vi "Launch_Async_Email.vi"() -> (0 "error out":errorcluster)   [LabVIEW 2018]
uses:
  Globals/Constants_global.vi
  Email_transfer_global.vi
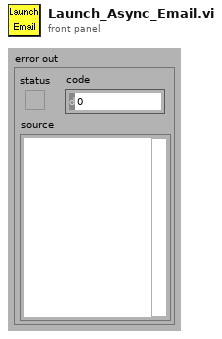
[diagram p1: front panel]
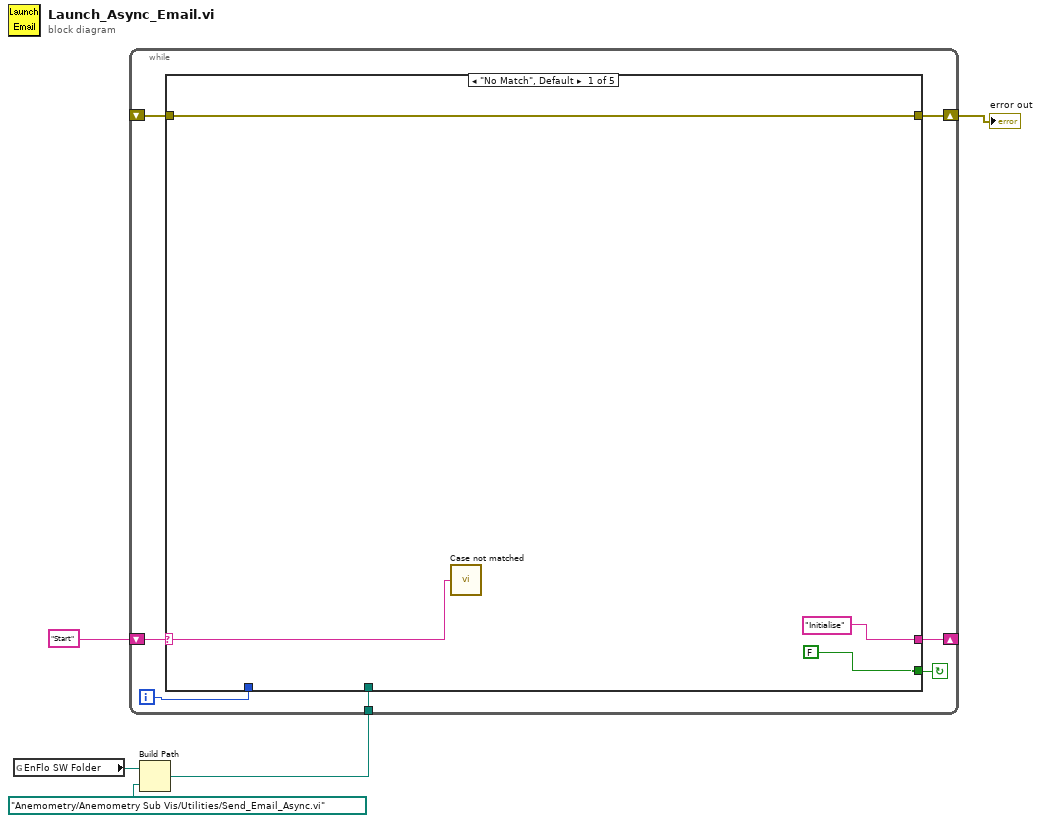
[diagram p0: block diagram]
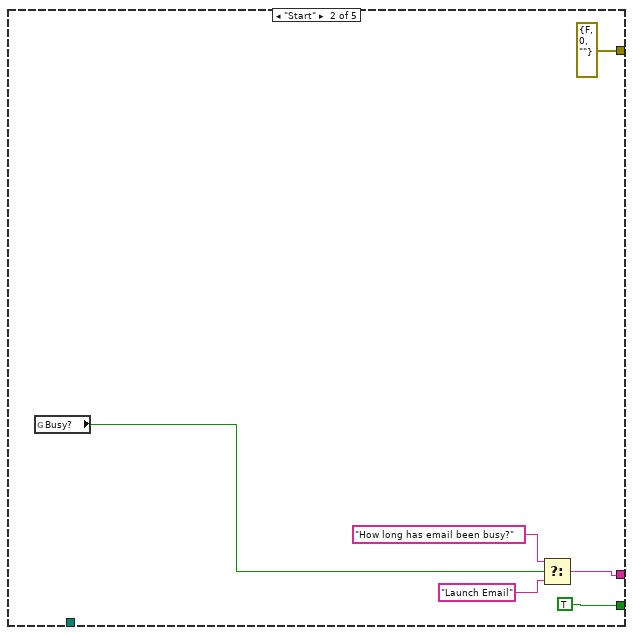
[diagram p2: hidden frame]
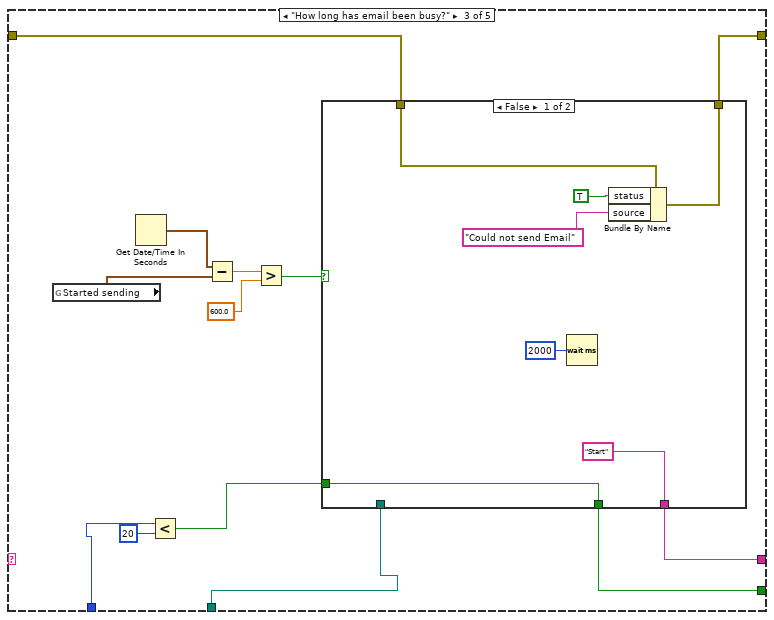
[diagram p3: hidden frame]
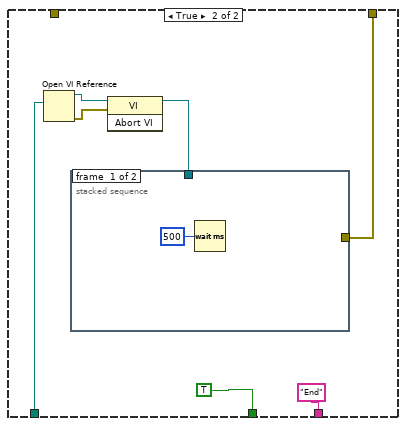
[diagram p4: hidden frame]
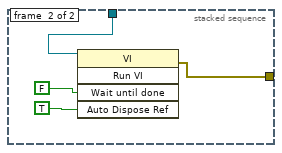
[diagram p5: hidden frame]
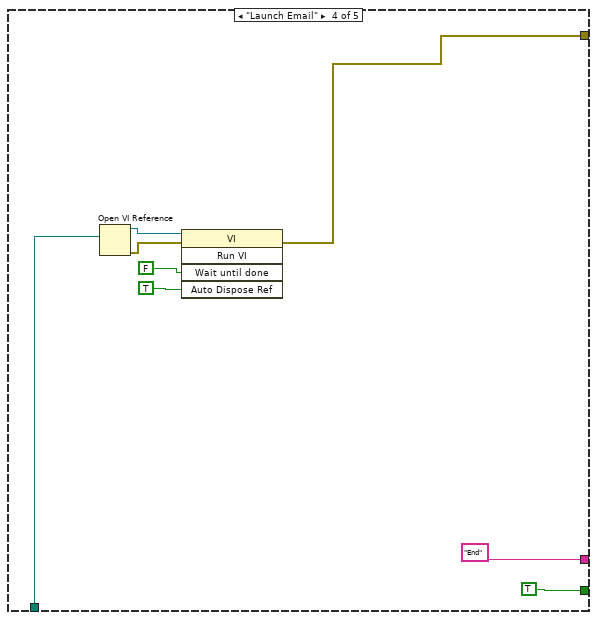
[diagram p6: hidden frame]
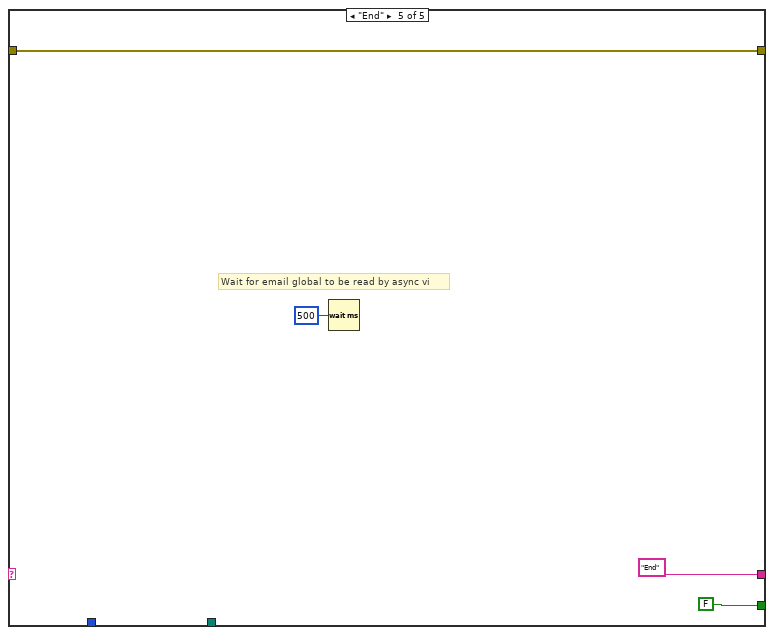
[diagram p7: hidden frame]
diagram:
  n1 = global read "Constants_global.vi" "EnFlo SW Folder"() -> (w3:path)
  n2 = Build Path(base path=w3, name or relative path=path "Anemometry/Anemometry Sub Vis/Utilities/Send_Email_Async.vi") -> (appended path=w2:path)
  n3 = while {
    shift-left: "Start" -> [w10]
    shift-right: [w11] -> _
    tunnel: w2 -> [w9]
    shift-right: [w8] -> w1
    shift-left: _ -> [w7]
    i -> [w6]
    stop <- w12 continue-if-true
    n4 = case shown="\"No Match\", Default" w10 {
      selector: w10 -> [w13 _ _ _ _]
      tunnel: [FALSE TRUE w28 TRUE FALSE] -> w12
      tunnel: ["Initialise" w18 w29 "End" "End"] -> w11
      tunnel: w9 -> [_ _ w30 w56 _]
      tunnel: [w14 errorcluster {"status"=FALSE, "code"=0, "source"=""} ("error out") w24 w55 w63] -> w8
      tunnel: w7 -> [w14 _ w23 _ w63]
      tunnel: w6 -> [_ _ w27 _ _]
      frame "No Match", Default {
        n5 = call "Case not matched.vi"("Case Name not Matched"=w13) -> ()
      }
      frame "Start" {
        n6 = global read "Email_transfer_global.vi" "Busy?"() -> (w20:bool)
        n7 = Select(t="How long has email been busy?", s=w20, f="Launch Email") -> (s? t:f=w18:string)
      }
      frame "How long has email been busy?" {
        n8 = global read "Email_transfer_global.vi" "Started sending"() -> (w34:timestamp)
        n9 = Get Date/Time In Seconds() -> (seconds since 1Jan1904=w35:timestamp)
        n10 = Less?(x=w27, y=20) -> (x < y?=w25:bool)
        n11 = Subtract(x=w35, y=w34) -> (x-y=w33:dbl)
        n12 = Greater?(x=w33, y=600.0) -> (0:w31:bool)
        n13 = case shown="False" w31 {
          tunnel: w30 -> [_ w47]
          tunnel: ["Start" "End"] -> w29
          tunnel: [w40 TRUE] -> w28
          tunnel: w25 -> [w40 _]
          tunnel: [w38 w44] -> w24
          tunnel: w23 -> [w39 _]
          frame False {
            n14 = Wait (ms)(milliseconds to wait=u32 2000) -> ()  [unwired: 1 out]
            n15 = Bundle By Name(cluster=w39, "status"=TRUE, "source"="Could not send Email") -> (w38:errorcluster)
          }
          frame True {
            n16 = Open VI Reference(vi path=w47) -> (vi reference=w48:refnum<vi>, error out=w49:errorcluster)  [unwired: 1 in, 4 out]
            n17 = invoke class="VI" method="Abort VI"(reference=w48, error in=w49) -> (reference out=w43:refnum<vi>)  [unwired: 1 in, 2 out]
            n18 = stacked-sequence {
              tunnel: [_ w51] -> w44
              tunnel: w43 -> [_ w52]
              frame #0 {
                n19 = Wait (ms)(milliseconds to wait=u32 500) -> ()  [unwired: 1 out]
              }
              frame #1 {
                n20 = invoke class="VI" method="Run VI"(reference=w52, "Wait until done"=FALSE, "Auto Dispose Ref"=TRUE) -> (error out=w51:errorcluster)  [unwired: 2 in, 4 out]
              }
            }
          }
        }
      }
      frame "Launch Email" {
        n21 = Open VI Reference(vi path=w56) -> (vi reference=w59:refnum<vi>, error out=w60:errorcluster)  [unwired: 1 in, 4 out]
        n22 = invoke class="VI" method="Run VI"(reference=w59, error in=w60, "Wait until done"=FALSE, "Auto Dispose Ref"=TRUE) -> (error out=w55:errorcluster)  [unwired: 1 in, 4 out]
      }
      frame "End" {
        # "Wait for email global to be read by async vi"
        n23 = Wait (ms)(milliseconds to wait=u32 500) -> ()  [unwired: 1 out]
      }
    }
  }
  "error out" <- w1
